vi "Cabration.vi"(9 "L_D 2":dbl, 10 "L_C 2":dbl, 11 "MainOption":T2={"Check Vacuum2-5"=FALSE, "No Press?"=FALSE, "Vibration Waiting Time(sec)"=0, "1 "=TRUE, "2"=TRUE, "3"=TRUE, "Devacuum"=FALSE, "Time1 ms"=0, "Time2 ms"=0, "check vacuum 1"=FALSE, "devacuum time when go up"=0.0, "Up (ms)"=0}) -> (1 "L_D":dbl, 2 "L_C":dbl)   [LabVIEW 2016, in "DIS_SubPannel.lvlib"]
uses:
  DISGradingMachine/SubPannel/DIS_SubPannel.lvlib
  DISGradingMachine/sub/MachineParType/MachineParType.ctl
  meter global.vi
panel:
  in  "Tab Control":enum32{"Page 1", "Page 2"}(tab)
  out "connectd":bool
  in  "stop":bool
  in  "cable":enum16{"0M", "1M", "2M"}(ring)=enum."2M"
  in  "int":bool
  in  "Range":T1(ring)
  in  "Frequencies":enum16{"120HZ", "1K  HZ", "1M HZ"}(ring)
  out "CAP cab":dbl format="%#_6p"
  out "DF  Cab":dbl
  in  "Trigger":bool
  out "G":dbl
  out "B":dbl
  out "R":dbl
  out "X":dbl
  in  "Trigger C":bool
  in  "Trigger S":bool
  in  "Trigger Load  write":bool
  in  "C":dbl
  in  "F 2":u16(ring)=2 items=["mF", "uF", "nF", "pF"]
  in  "D":dbl
  in  "Cmd_close":bool
  in  "Cmd_open":bool
  out "E4981 VISA resource name":refnum<visa-resource-name>
  out "String":string
  out "Label.Text":string
  in  "indexup 2":bool caption="Index Down"
  # "E4981A電錶校正"
  # "0 m When you do not use the test lead (in other words, when you connect\nthe test fixture directly to the UNKNOWN terminal).\n1 m When you use the Agilent 16048A/B Agilent test lead.\n2 m When you use the Agilent 16048D test lead."
  # "OPEN"
  # "SHORT"
  # "LOAD read"
  # "LOAD"
  # "機台參數"
  # "電錶1 電性測試"
  # "電錶2  TV   耐壓測試"
  # "電錶3  IR 絕緣阻抗測試"
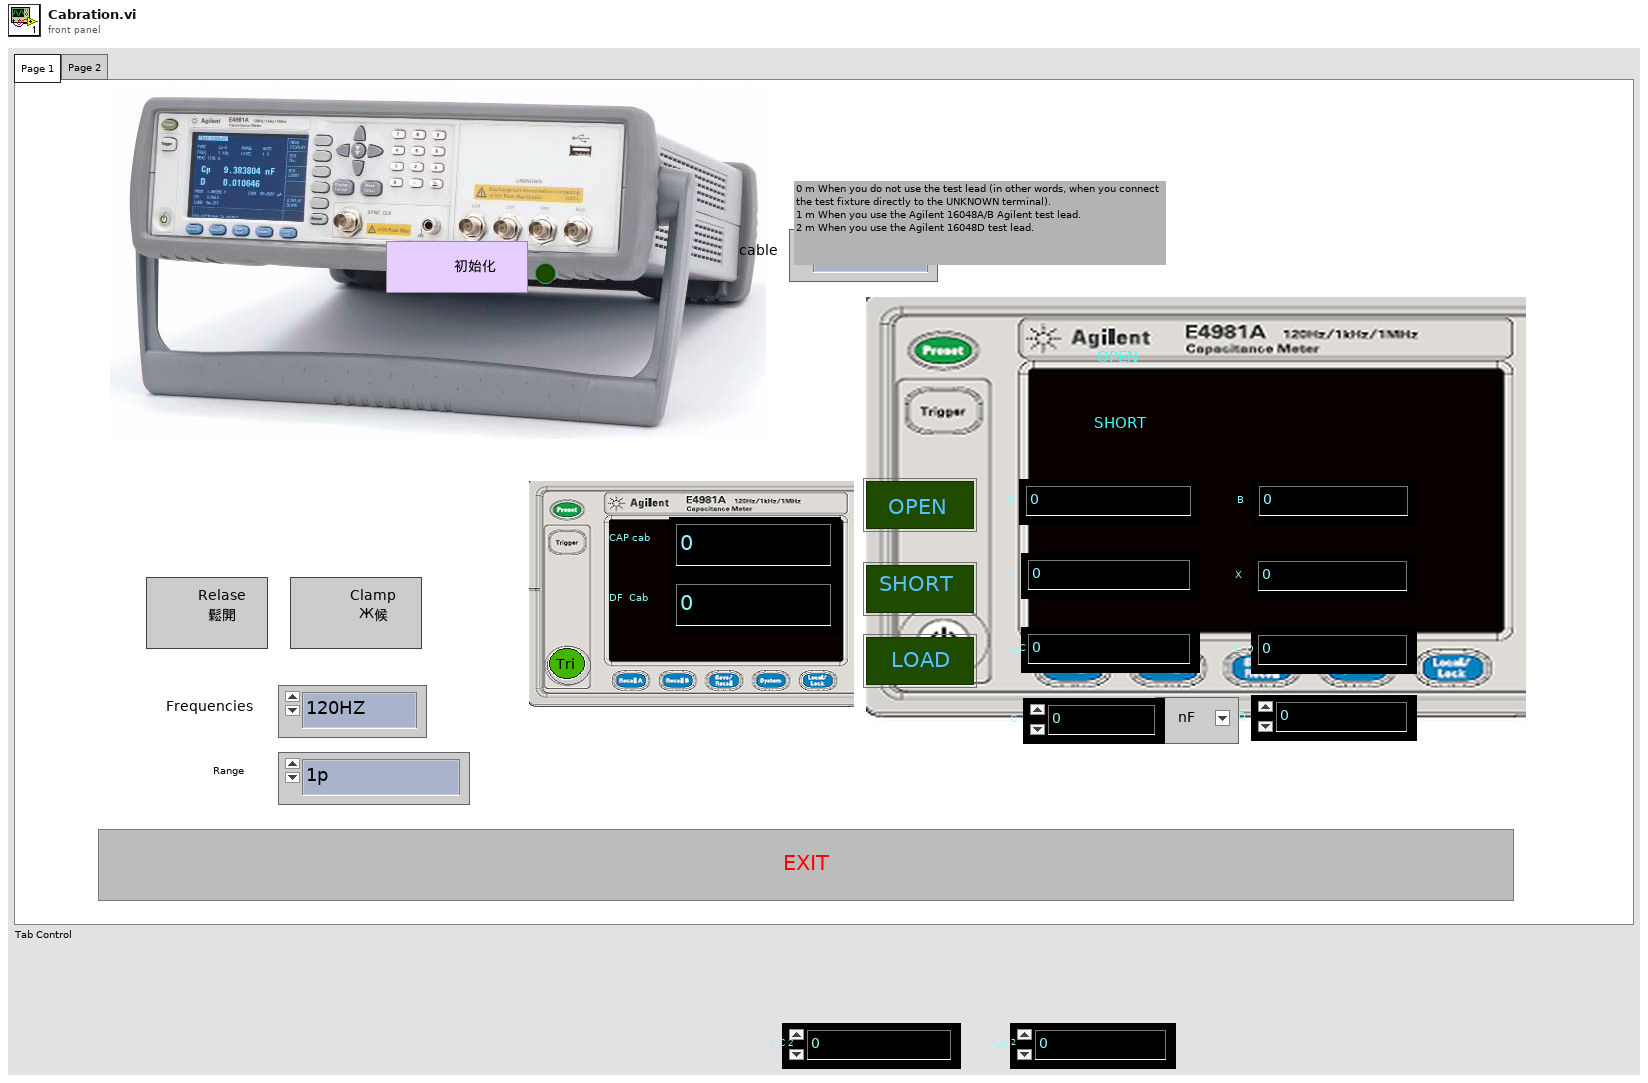
[diagram p1: front panel]
types:
  T1 = enum16{"1p", "2.2p", "4.7p", "10p", "22p", "47p", "100p", "220p", "470p", "1n", "2.2n", "4.7n", "10n", "22n", "47n", "100n", "220n", "470n", "1u", "2.2u", "4.7u", "10u", "22u", "47u", "100u", "220u", "470u", "1m", "AUTO", ""}
  T2 = typedef "MachineParType.ctl" = cluster{"Check Vacuum2-5":bool, "No Press?":bool, "Vibration Waiting Time(sec)":u32, "1 ":bool, "2":bool, "3":bool, "Devacuum":bool, "Time1 ms":u32, "Time2 ms":u32, "check vacuum 1":bool, "devacuum time when go up":dbl, "Up (ms)":u32}
  T3 = typedef "TypeDef_PNData.ctl" = cluster{"External Diameter":dbl, "Height":dbl, "Range":enum16{"1p", "2.2p", "4.7p", "10p", "22p", "47p", "100p", "220p", "470p", "1n", "2.2n", "4.7n", "10n", "22n", "47n", "100n", "220n", "470n", "1u", "2.2u", "4.7u", "10u", "22u", "47u", "100u", "220u", "470u", "1m", "AUTO", ""}, "DFmin":dbl, "Cap_num":dbl, "F":u16, "BIN3+":dbl, "BIN3- ":dbl, "BIN2+":dbl, "BIN2-":dbl, "BIN1+":dbl, "BIN1-":dbl, "Frequencies":enum16{"120HZ", "1K  HZ", "1M HZ"}, "DFmax":dbl, "Part_5":dbl, "Part_6":dbl, "Part_4":dbl, "Part_8":dbl, "Part_7":dbl, "Par_2":dbl, "part_1":enum16{"DC", "AC"}, "Part_9":dbl, "Part_18":dbl, "Part_15":dbl, "Part_13":dbl, "Part_14":dbl, "Part_16":dbl, "Internal Diameter":dbl, "Part_14 (IR Max)":dbl}
  T4 = enum16{"Default0", "checkconnect", "int", "changeFEQ", "changeRange"}
  T5 = cluster{"Frequency (1:1kHz)":u16, "Frequency Shift (2: 0%)":u16, "Range":enum16{"1p", "2.2p", "4.7p", "10p", "22p", "47p", "100p", "220p", "470p", "1n", "2.2n", "4.7n", "10n", "22n", "47n", "100n", "220n", "470n", "1u", "2.2u", "4.7u", "10u", "22u", "47u", "100u", "220u", "470u", "1m", "AUTO", ""}}
  T6 = enum16{"Default0", "checkconnect", "int", "changeFEQ", "changeRange", "trigger"}
  T7 = cluster{"connectd":bool, "CAP cab":dbl, "DF  Cab":dbl}
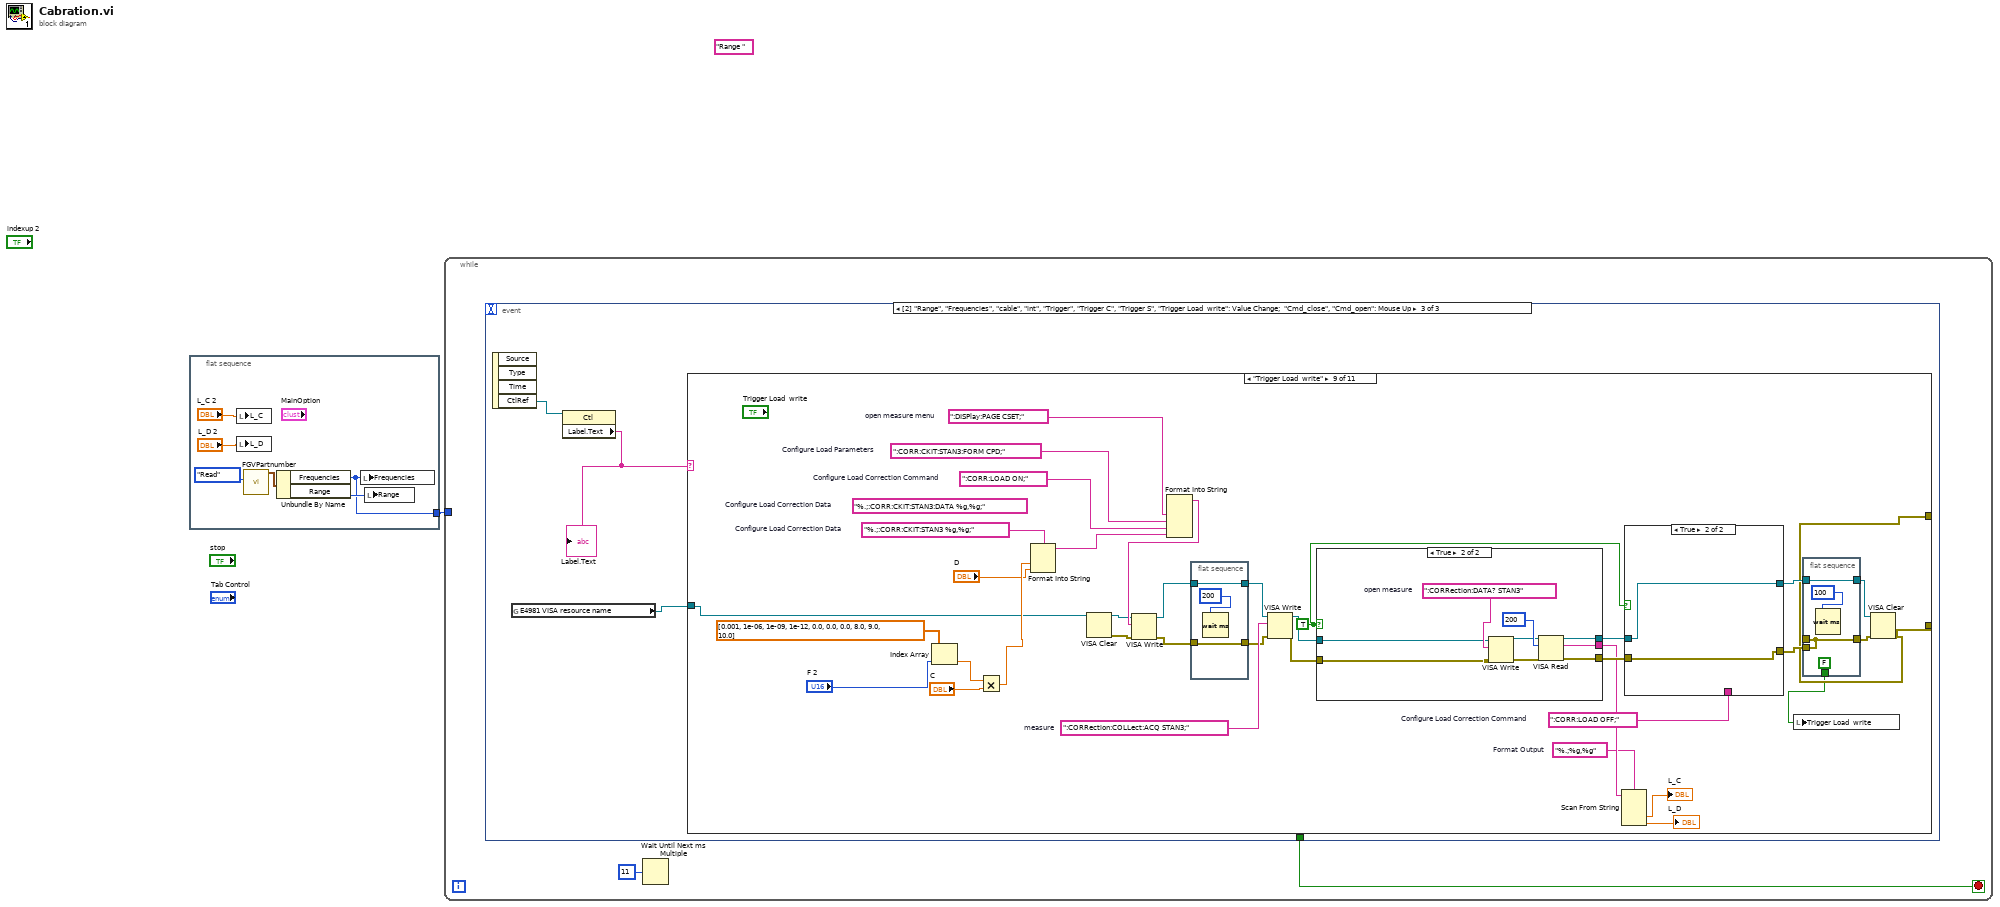
[diagram p0: block diagram]
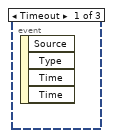
[diagram p2: hidden frame]
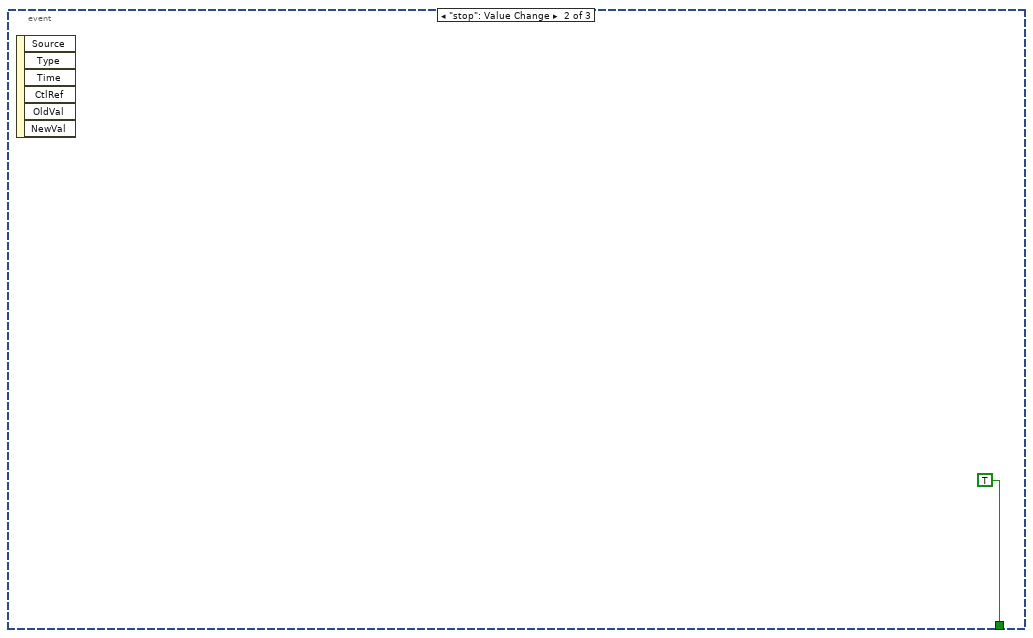
[diagram p3: hidden frame]
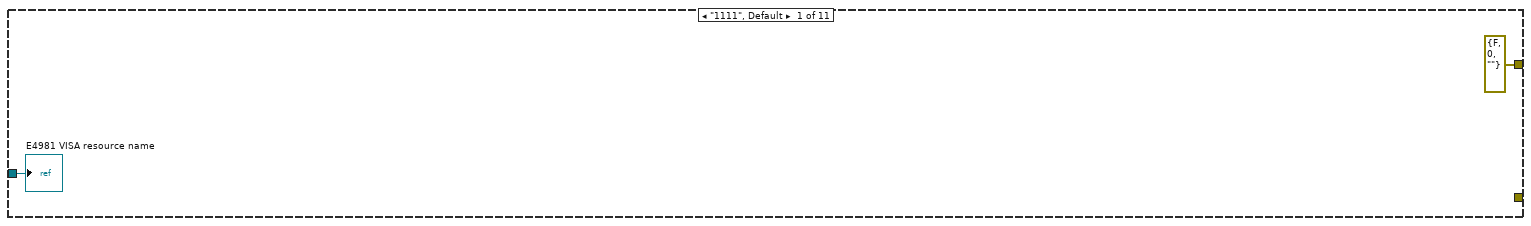
[diagram p4: hidden frame]
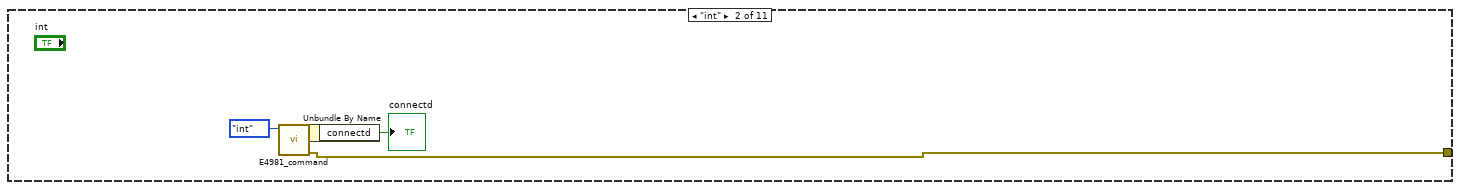
[diagram p5: hidden frame]
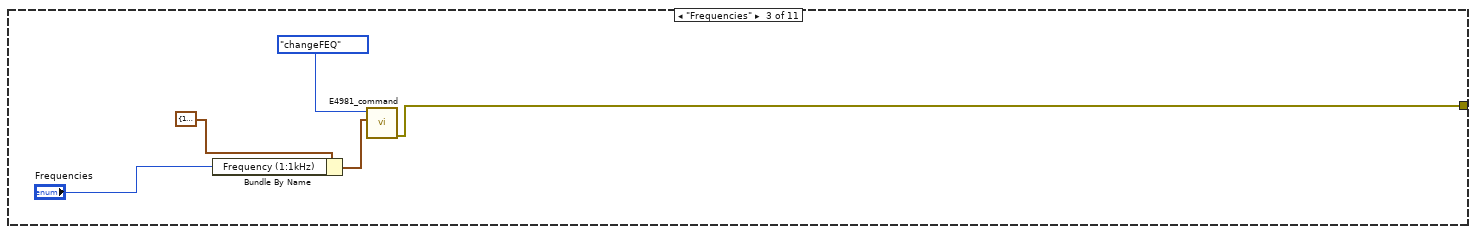
[diagram p6: hidden frame]
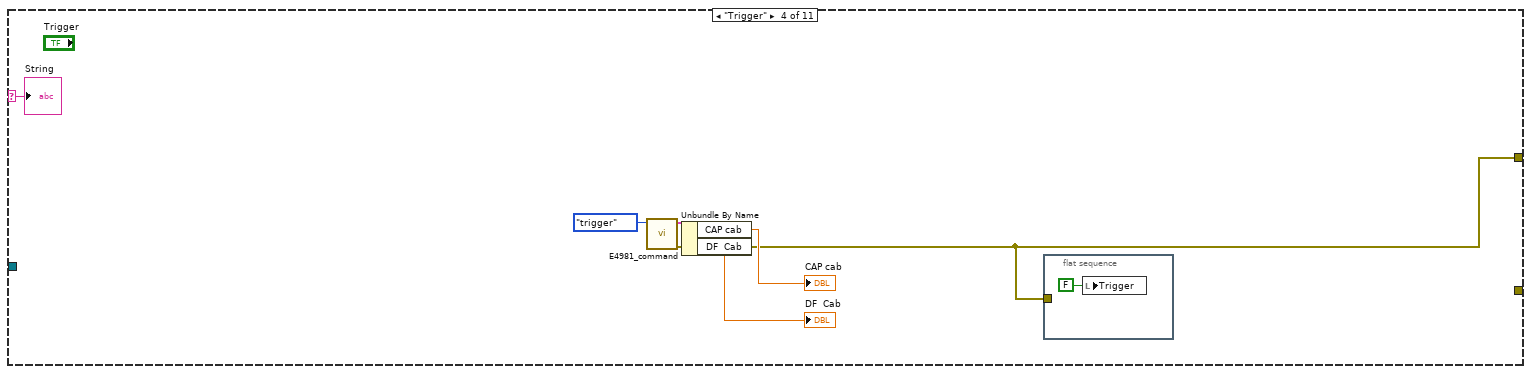
[diagram p7: hidden frame]
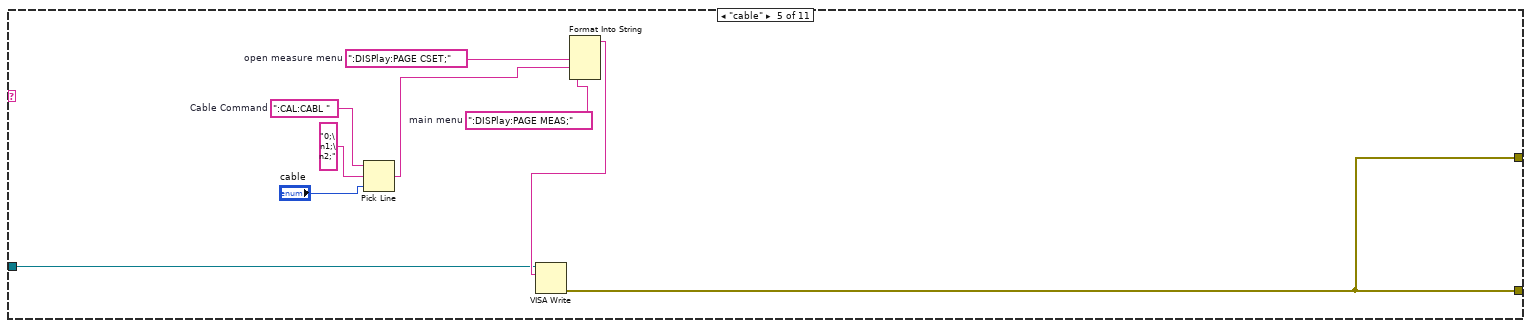
[diagram p8: hidden frame]
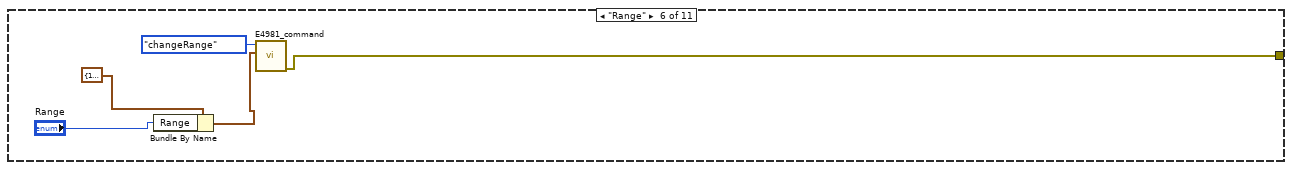
[diagram p9: hidden frame]
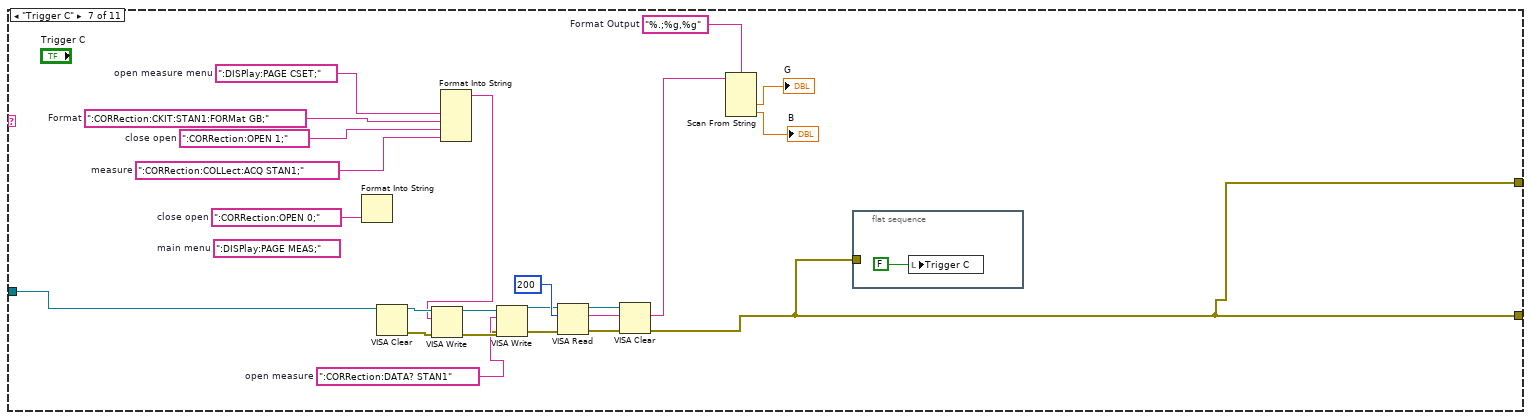
[diagram p10: hidden frame]
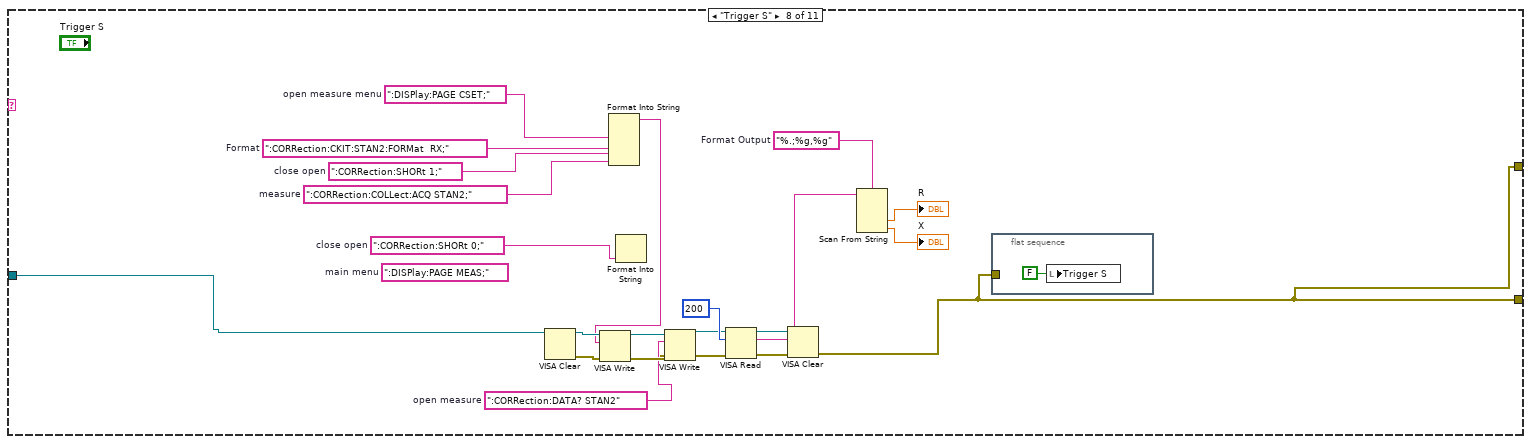
[diagram p11: hidden frame]
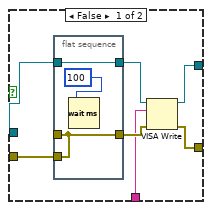
[diagram p12: hidden frame]
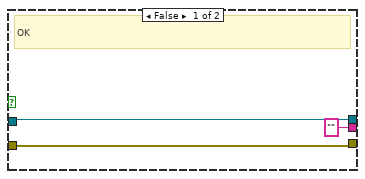
[diagram p13: hidden frame]
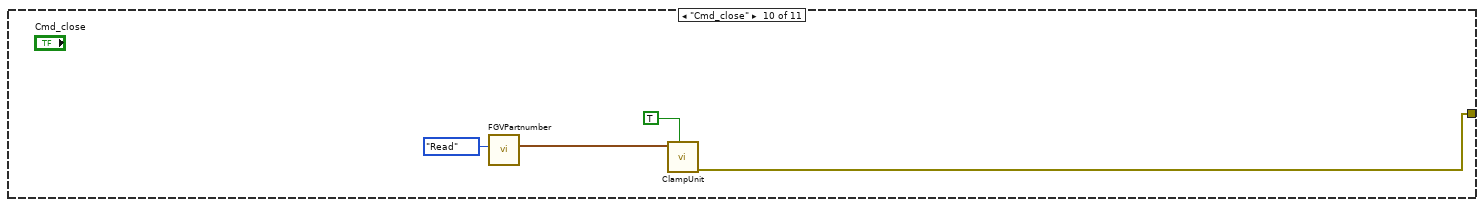
[diagram p14: hidden frame]
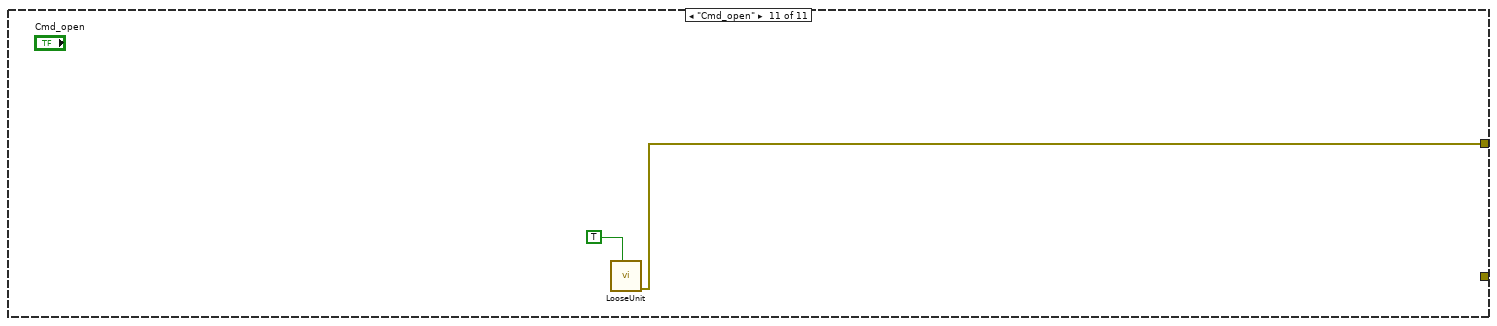
[diagram p15: hidden frame]
diagram:
  (unwired) "Range " ("Label.Text 2")
  n1 = flat-sequence {
    tunnel: [w4] -> w1
    frame #0 {
      n2 = local write "L_C"("L_C 2") -> ()
      n3 = local write "L_D"("L_D 2") -> ()
      n4 = call "FGVPartnumber.vi"("Enum"=enum16{"Write", "Read"}."Read") -> ("UnitParamiterCluster out"=w6:T3)  [unwired: 10 in]
      n5 = Unbundle By Name(w6) -> ("Frequencies"=w4:enum16{"120HZ", "1K  HZ", "1M HZ"}, "Range"=w5:T1)
      n6 = local write "Frequencies"(w4) -> ()
      n7 = local write "Range"(w5) -> ()
    }
  }
  n8 = while {
    tunnel: w1 -> [_]
    stop <- w9 stop-if-true
    n9 = event shown="[2] \"Range\", \"Frequencies\", \"cable\", \"int\", \"Trigger\", \"Trigger C\", \"Trigger S\", \"Trigger Load  write\": Value Change;  \"Cmd_close\", \"Cmd_open\": Mouse Up" {
      selector: _ -> [_ _ _]
      dyn-events: _ -> [_ _ _]
      timeout: _ -> [_ _ _]
      tunnel: [_ TRUE _] -> w9
      event Timeout {
        n10 = event-data() -> ()  [unwired: 1 in, 4 out]
      }
      event "stop": Value Change {
        n11 = event-data() -> ()  [unwired: 1 in, 6 out]
      }
      event "Range", "Frequencies", "cable", "int", "Trigger", "Trigger C", "Trigger S", "Trigger Load  write": Value Change; "Cmd_close", "Cmd_open": Mouse Up {
        n12 = event-data() -> ("CtlRef"=w13:refnum<vi>)  [unwired: 1 in, 3 out]
        n13 = global read "meter global.vi" "E4981 VISA resource name"() -> (w11:refnum<visa-resource-name>)
        n14 = property class="Ctl"(reference=w13) -> ("Label.Text"=w12:string)  [unwired: 1 in, 2 out]
        "Label.Text" <- w12
        n15 = case shown="\"Trigger Load  write\"" w12 {
          selector: w12 -> [_ _ _ w26 _ _ _ _ _ _ _]
          tunnel: [_ _ _ _ w32 _ w46 w69 w93 _ _] -> _
          tunnel: w11 -> [w15 _ _ _ w33 _ w49 w72 w94 _ _]
          tunnel: [errorcluster {"status"=FALSE, "code"=0, "source"=""} ("error out") w16 w20 w25 w32 w41 w46 w69 w93 w161 w163] -> _
          frame "1111", Default {
            "E4981 VISA resource name" <- w15
          }
          frame "int" {
            n16 = call "E4981_command.vi"("command"=T4."int") -> ("error out"=w16:errorcluster, "output"=w18:T7)  [unwired: 8 in, 1 out]
            n17 = Unbundle By Name(w18) -> ("connectd"=→"connectd":bool)
          }
          frame "Frequencies" {
            n18 = Bundle By Name(cluster=T5 {"Frequency (1:1kHz)"=1, "Frequency Shift (2: 0%)"=2, "Range"=enum."1p"} ("input"), "Frequency (1:1kHz)"="Frequencies") -> (w21:T5)
            n19 = call "E4981_command.vi"("input"=w21, "command"=T4."changeFEQ") -> ("error out"=w20:errorcluster)  [unwired: 7 in, 2 out]
          }
          frame "Trigger" {
            n20 = call "E4981_command.vi"("command"=T6."trigger") -> ("error out"=w25:errorcluster, "output"=w29:T7)  [unwired: 8 in, 1 out]
            n21 = Unbundle By Name(w29) -> ("CAP cab"=→"CAP cab":dbl, "DF  Cab"=→"DF  Cab":dbl)
            n22 = flat-sequence {
              tunnel: w25 -> [_]
              frame #0 {
                n23 = local write "Trigger"(FALSE ("Trigger")) -> ()
              }
            }
            "String" <- w26
          }
          frame "cable" {
            w35 = ":DISPlay:PAGE MEAS;"  # main menu
            w38 = ":DISPlay:PAGE CSET;"  # open measure menu
            w39 = ":CAL:CABL "  # Cable Command
            n24 = Pick Line(string ("")=w39, multi-line string="0;\n1;\n2;", line index="cable") -> (output string=w37:string)
            n25 = Format Into String(w38, w37, w35) -> (resulting string=w36:string)  [unwired: 3 in, 1 out]
            n26 = VISA Write(VISA resource name=w33, write buffer=w36) -> (error out=w32:errorcluster)  [unwired: 1 in, 2 out]
          }
          frame "Range" {
            n27 = Bundle By Name(cluster=T5 {"Frequency (1:1kHz)"=1, "Frequency Shift (2: 0%)"=2, "Range"=enum."1p"} ("input"), "Range"="Range") -> (w43:T5)
            n28 = call "E4981_command.vi"("input"=w43, "command"=T4."changeRange") -> ("error out"=w41:errorcluster)  [unwired: 7 in, 2 out]
          }
          frame "Trigger C" {
            w50 = ":CORRection:OPEN 1;"  # close open
            w56 = "%.;%g,%g"  # Format Output
            w61 = ":CORRection:DATA? STAN1"  # open measure
            w66 = ":CORRection:OPEN 0;"  # close open
            w67 = ":CORRection:COLLect:ACQ STAN1;"  # measure
            w51 = ":CORRection:CKIT:STAN1:FORMat GB;"  # Format
            (unwired) ":DISPlay:PAGE MEAS;"  # main menu
            w52 = ":DISPlay:PAGE CSET;"  # open measure menu
            n29 = Format Into String(w66) -> ()  [unwired: 3 in, 2 out]
            n30 = VISA Clear(VISA resource name=w49) -> (VISA resource name out=w65:refnum<visa-resource-name>, error out=w64:errorcluster)  [unwired: 1 in]
            n31 = Format Into String(w52, w51, w50, w67) -> (resulting string=w57:string)  [unwired: 3 in, 1 out]
            n32 = VISA Write(VISA resource name=w65, write buffer=w57, error in (no error)=w64) -> (VISA resource name out=w63:refnum<visa-resource-name>, error out=w62:errorcluster)  [unwired: 1 out]
            n33 = VISA Write(VISA resource name=w63, write buffer=w61, error in (no error)=w62) -> (VISA resource name out=w58:refnum<visa-resource-name>, error out=w59:errorcluster)  [unwired: 1 out]
            n34 = VISA Read(VISA resource name=w58, byte count=u32 200, error in (no error)=w59) -> (VISA resource name out=w54:refnum<visa-resource-name>, read buffer=w55:string, error out=w53:errorcluster)  [unwired: 1 out]
            n35 = VISA Clear(VISA resource name=w54, error in (no error)=w53) -> (error out=w46:errorcluster)  [unwired: 1 out]
            n36 = Scan From String(format string=w56, input string=w55) -> (output 1=→"G":dbl, output 2=→"B":dbl)  [unwired: 4 in, 3 out]
            n37 = flat-sequence {
              tunnel: w46 -> [_]
              frame #0 {
                n38 = local write "Trigger C"(FALSE) -> ()
              }
            }
          }
          frame "Trigger S" {
            w74 = ":CORRection:SHORt 1;"  # close open
            w79 = "%.;%g,%g"  # Format Output
            w84 = ":CORRection:DATA? STAN2"  # open measure
            w89 = ":CORRection:SHORt 0;"  # close open
            w90 = ":CORRection:COLLect:ACQ STAN2;"  # measure
            w73 = ":CORRection:CKIT:STAN2:FORMat  RX;"  # Format
            (unwired) ":DISPlay:PAGE MEAS;"  # main menu
            w75 = ":DISPlay:PAGE CSET;"  # open measure menu
            n39 = VISA Clear(VISA resource name=w72) -> (VISA resource name out=w88:refnum<visa-resource-name>, error out=w87:errorcluster)  [unwired: 1 in]
            n40 = Format Into String(w75, w73, w74, w90) -> (resulting string=w80:string)  [unwired: 3 in, 1 out]
            n41 = VISA Write(VISA resource name=w88, write buffer=w80, error in (no error)=w87) -> (VISA resource name out=w86:refnum<visa-resource-name>, error out=w85:errorcluster)  [unwired: 1 out]
            n42 = Format Into String(w89) -> ()  [unwired: 3 in, 2 out]
            n43 = VISA Write(VISA resource name=w86, write buffer=w84, error in (no error)=w85) -> (VISA resource name out=w81:refnum<visa-resource-name>, error out=w82:errorcluster)  [unwired: 1 out]
            n44 = VISA Read(VISA resource name=w81, byte count=u32 200, error in (no error)=w82) -> (VISA resource name out=w77:refnum<visa-resource-name>, read buffer=w78:string, error out=w76:errorcluster)  [unwired: 1 out]
            n45 = VISA Clear(VISA resource name=w77, error in (no error)=w76) -> (error out=w69:errorcluster)  [unwired: 1 out]
            n46 = Scan From String(format string=w79, input string=w78) -> (output 1=→"R":dbl, output 2=→"X":dbl)  [unwired: 4 in, 3 out]
            n47 = flat-sequence {
              tunnel: w69 -> [_]
              frame #0 {
                n48 = local write "Trigger S"(FALSE ("Trigger S")) -> ()
              }
            }
          }
          frame "Trigger Load  write" {
            w123 = TRUE
            w117 = "%.;%g,%g"  # Format Output
            w113 = ":CORR:LOAD OFF;"  # Configure Load Correction Command
            (unwired) "%.;:CORR:CKIT:STAN3:DATA %g,%g;"  # Configure Load Correction Data
            w116 = "%.;:CORR:CKIT:STAN3 %g,%g;"  # Configure Load Correction Data
            w108 = ":CORRection:COLLect:ACQ STAN3;"  # measure
            w115 = ":CORR:LOAD ON;"  # Configure Load Correction Command
            w101 = ":DISPlay:PAGE CSET;"  # open measure menu
            w102 = ":CORR:CKIT:STAN3:FORM CPD;"  # Configure Load Parameters
            n49 = Index Array(array=dbl[] [0.001, 1e-06, 1e-09, 1e-12, 0.0, 0.0, 0.0, 8.0, 9.0, 10.0] ("box"), index="F 2") -> (element=w96:dbl)
            n50 = Multiply(x=w96, y="C") -> (x*y=w125:dbl)
            n51 = Format Into String(format string=w116, w125, "D") -> (resulting string=w114:string)  [unwired: 2 in, 1 out]
            n52 = VISA Clear(VISA resource name=w94) -> (VISA resource name out=w99:refnum<visa-resource-name>, error out=w100:errorcluster)  [unwired: 1 in]
            n53 = Format Into String(w101, w102, w115, w114) -> (resulting string=w103:string)  [unwired: 3 in, 1 out]
            n54 = VISA Write(VISA resource name=w99, write buffer=w103, error in (no error)=w100) -> (VISA resource name out=w105:refnum<visa-resource-name>, error out=w106:errorcluster)  [unwired: 1 out]
            n55 = flat-sequence {
              tunnel: [w157] -> w104
              tunnel: w105 -> [w157]
              tunnel: w106 -> [w156]
              tunnel: [w156] -> w107
              frame #0 {
                n56 = Wait (ms)(milliseconds to wait=u32 200 ("byte count")) -> ()  [unwired: 1 out]
              }
            }
            n57 = VISA Write(VISA resource name=w104, write buffer=w108, error in (no error)=w107) -> (VISA resource name out=w120:refnum<visa-resource-name>, error out=w121:errorcluster)  [unwired: 1 out]
            n58 = case shown="True" w123 {
              tunnel: ["" ("read buffer") w147] -> w118
              tunnel: [w142 w146] -> w119
              tunnel: w120 -> [w142 w145]
              tunnel: w121 -> [w141 w144]
              tunnel: [w141 w143] -> w122
              frame False {
                # "OK"
              }
              frame True {
                w151 = ":CORRection:DATA? STAN3"  # open measure
                n59 = VISA Write(VISA resource name=w145, write buffer=w151, error in (no error)=w144) -> (VISA resource name out=w148:refnum<visa-resource-name>, error out=w149:errorcluster)  [unwired: 1 out]
                n60 = VISA Read(VISA resource name=w148, byte count=u32 200, error in (no error)=w149) -> (VISA resource name out=w146:refnum<visa-resource-name>, read buffer=w147:string, error out=w143:errorcluster)  [unwired: 1 out]
              }
            }
            n61 = Scan From String(format string=w117, input string=w118) -> (output 1=→"L_C":dbl, output 2=→"L_D":dbl)  [unwired: 4 in, 3 out]
            n62 = case shown="True" w123 {
              tunnel: [w132 w139] -> w109
              tunnel: [w131 w138] -> w111
              tunnel: w113 -> [w130 _]
              tunnel: w119 -> [w129 w139]
              tunnel: w122 -> [w128 w138]
              frame False {
                n63 = flat-sequence {
                  tunnel: [w136] -> w133
                  tunnel: w129 -> [w136]
                  tunnel: [w135] -> _
                  tunnel: [w135] -> w134
                  tunnel: w128 -> [w135]
                  frame #0 {
                    n64 = Wait (ms)(milliseconds to wait=u32 100 ("byte count")) -> ()  [unwired: 1 out]
                  }
                }
                n65 = VISA Write(VISA resource name=w133, write buffer=w130, error in (no error)=w134) -> (VISA resource name out=w132:refnum<visa-resource-name>, error out=w131:errorcluster)  [unwired: 1 out]
              }
              frame True {
              }
            }
            n66 = local write "Trigger Load  write"(w92) -> ()
            n67 = flat-sequence {
              tunnel: [w154] -> w110
              tunnel: w109 -> [w154]
              tunnel: [w153] -> _
              tunnel: [w153] -> w112
              tunnel: w111 -> [w153]
              tunnel: [FALSE] -> w92
              frame #0 {
                n68 = Wait (ms)(milliseconds to wait=u32 100 ("byte count")) -> ()  [unwired: 1 out]
              }
            }
            n69 = VISA Clear(VISA resource name=w110, error in (no error)=w112) -> (error out=w93:errorcluster)  [unwired: 1 out]
          }
          frame "Cmd_close" {
            n70 = call "FGVPartnumber.vi"("Enum"=enum16{"Write", "Read"}."Read") -> ("UnitParamiterCluster out"=w159:T3)  [unwired: 10 in]
            n71 = call "ClampUnit.vi"("SkipWaitStep?"=TRUE, "UnitParamiterCluster out"=w159) -> ("error out"=w161:errorcluster)  [unwired: 9 in]
          }
          frame "Cmd_open" {
            n72 = call "LooseUnit.vi"("SkipWaitStep?"=TRUE) -> ("error out"=w163:errorcluster)  [unwired: 10 in]
          }
        }
      }
    }
    n73 = Wait Until Next ms Multiple(millisecond multiple=u32 11) -> ()  [unwired: 1 out]
  }
